vi "Write Message Data.lvclass.vi"(8 "error in (no error)":errorcluster, 10 "Message Data.lvclass":refnum<class "Message Data.lvclass">, 11 "Message Type in":refnum<class "Message Type.lvclass">) -> (0 "error out":errorcluster, 3 "Message Type out":refnum<class "Message Type.lvclass">)   [LabVIEW 2023, in "Message Type.lvclass"]
uses:
  Message Type.lvclass
  Message Type.lvclass/Message Type.ctl
  Message Data/Message Data.lvclass
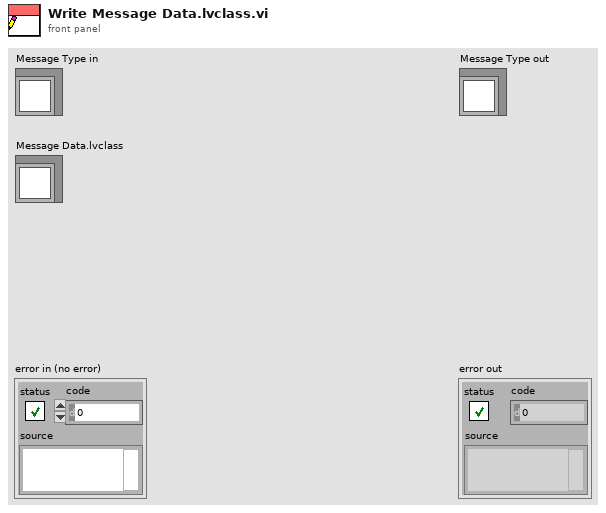
[diagram p1: front panel]
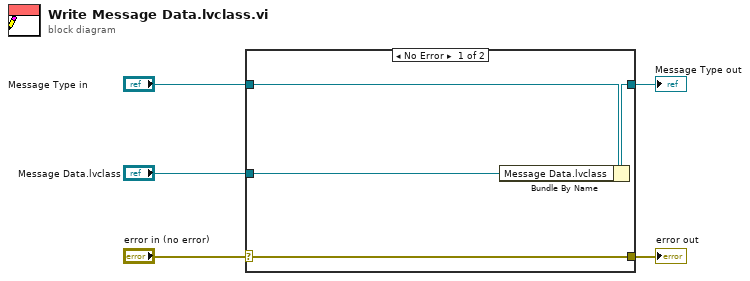
[diagram p0: block diagram]
diagram:
  n1 = case shown="No Error" "error in (no error)" {
    selector: "error in (no error)" -> [w9 w10]
    tunnel: [w9 w10] -> w4
    tunnel: [w7 w11] -> w2
    tunnel: "Message Type in" -> [w8 w11]
    tunnel: "Message Data.lvclass" -> [w6 _]
    frame No Error {
      n2 = Bundle By Name(cluster=w8, "Message Data.lvclass"=w6) -> (w7:refnum<class "Message Type.lvclass">)
    }
    frame Error {
    }
  }
  "error out" <- w4
  "Message Type out" <- w2
